vi "CCC Example - Client.vi"() -> ()   [LabVIEW 2010]
doc: "This VI shows an example of how to use the CVT Client Communication API. This VI is meant to be used in conjunction with \"CCC Server Example.vi\"."
uses:
  vi.lib/NI/CCC/Tag Configuration.ctl
  <vilib>/NI/Current Value Table/Type Defs/Data Types.ctl
  vi.lib/NI/CCC/Tag Direction.ctl
  <vilib>/NI/Current Value Table/Type Defs/Single Tag.ctl
  <vilib>/NI/Current Value Table/Type Defs/File Format.ctl
  <vilib>/NI/Current Value Table/Type Defs/Tag Grouping set.ctl
  <vilib>/NI/Current Value Table/DataTypes/Double_Write.vi
  <vilib>/NI/Current Value Table/DataTypes/String_Write.vi
  <vilib>/NI/Current Value Table/DataTypes/Double_Read.vi
  <vilib>/NI/Current Value Table/DataTypes/Boolean_Read.vi
  <vilib>/NI/Current Value Table/Type to Enum.vi
  <vilib>/NI/Current Value Table/DataTypes/Double_Type To Enum.vi
  <vilib>/NI/Current Value Table/DataTypes/String_Type To Enum.vi
  <vilib>/NI/Current Value Table/DataTypes/Boolean_Type To Enum.vi
  <vilib>/NI/Current Value Table/FGVs/CVT Globals.vi
  <vilib>/NI/Current Value Table/FGVs/Tag Memory.vi
  <vilib>/NI/Current Value Table/Memory Block.vi
  <vilib>/NI/Current Value Table/DataTypes/Double_Memory Block.vi
  <vilib>/NI/Current Value Table/DataTypes/String_Memory Block.vi
  <vilib>/NI/Current Value Table/DataTypes/Boolean_Memory Block.vi
  vi.lib/NI/CCC/NI_CCC.lvlib
  <vilib>/NI/Current Value Table/Current Value Table.lvlib
panel:
  in  "Tab Control":enum32{"Tag Configuration", "Program Operation"}(tab)=enum."Program Operation"
  in  "CVT Tags":T1[](array[typedef])=[{"Data Type"=enum."Double", "Name"="Input1", "Value"="", "Description"=""}, {"Data Type"=enum."Double", "Name"="Input2", "Value"="", "Description"=""}, {"Data Type"=enum."Double", "Name"="Output", "Value"="", "Description"=""}, {"Data Type"=enum."String", "Name"="Operation", "Value"="", "Description"=""}, {"Data Type"=enum."Boolean", "Name"="ClientError", "Value"="", "Description"=""}]
  in  "CCC Tags":T3[](array[typedef])=[{"name"="Input1", "data type"=enum."Double", "direction"=enum."Write", "bound address"="Float1"}, {"name"="Input2", "data type"=enum."Double", "direction"=enum."Write", "bound address"="Float2"}, {"name"="Output", "data type"=enum."Double", "direction"=enum."Read", "bound address"="Float3"}, {"name"="Operation", "data type"=enum."String", "direction"=enum."Write", "bound address"="Operand"}, {"name"="ClientError", "data type"=enum."Boolean", "direction"=enum."Read", "bound address"="Error"}]
  in  "Server IP Address":string="0.0.0.0"
  in  "Input1":dbl=4.0
  in  "Input2":dbl=2.0
  in  "Operation":string="Add" caption="Choose from:\nAdd, Subtract, Multiply, Divide"
  in  "stop":bool
  out "Output":dbl
  out "Error":bool
  # "Directions:\nRun \"CCC Example - Server.vi\" first, then run this VI."
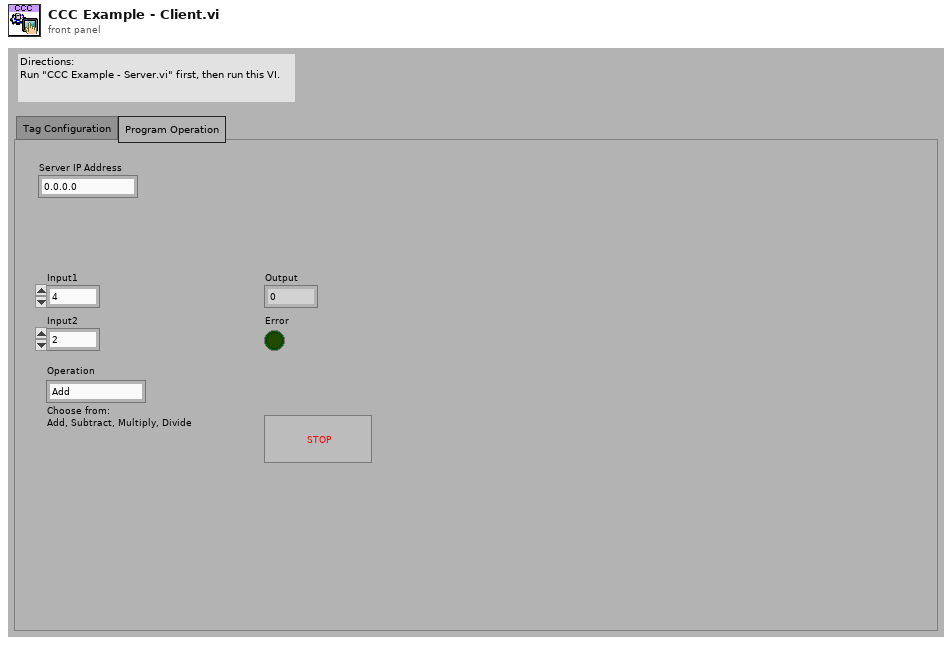
[diagram p1: front panel]
types:
  T1 = typedef "Current Value Table.lvlib/Single Tag.ctl" = cluster{"Data Type":T2, "Name":string, "Value":string, "Description":string}
  T2 = typedef "Current Value Table.lvlib/Data Types.ctl" = enum16{"Double", "Single", "I64", "I32", "I16", "I8", "U64", "U32", "U16", "U8", "String", "Boolean", "Array of U8", "Array of U16", "Array of U32", "Array of U64", "Array of I64", "Array of I32", "Array of I16", "Array of I8", "Array of Double", "Array of Single", "Array of Boolean", "Array of String"}
  T3 = typedef "NI_CCC.lvlib/Tag Configuration.ctl" = cluster{"name":string, "data type":T2, "direction":T4, "bound address":string}
  T4 = typedef "NI_CCC.lvlib/Tag Direction.ctl" = enum32{"<none>", "Read", "Write"}
  T5 = typedef "Current Value Table.lvlib/File Format.ctl" = cluster{"Tags":T1[], "Group Listings":T6[]}
  T6 = typedef "Current Value Table.lvlib/Tag Grouping set.ctl" = cluster{"Group":string, "Tag Names":string[]}
  T7 = typedef "NI_CCC.lvlib/Connection ID.ctl" = cluster{"server ID":string, "connection ID":T8, "meta data":T9[], "write tag list":T3[], "read tag list":T3[]}
  T8 = typedef "NI STM.lvlib/TCP Connection Info.ctl" = cluster{"connection ID":refnum<k5>, "Meta data":T9[]}
  T9 = typedef "NI STM.lvlib/MetaDataElement.ctl" = string
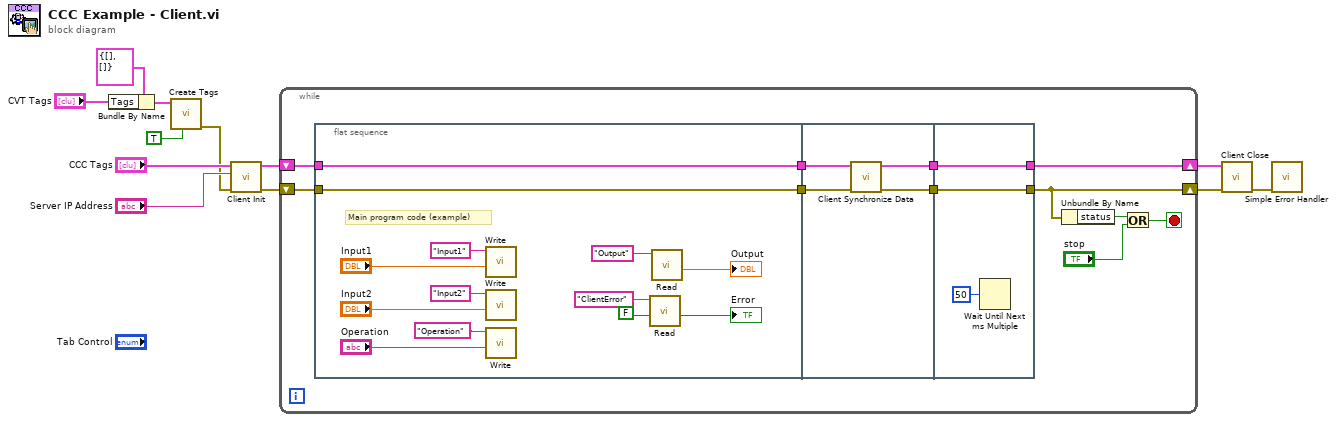
[diagram p0: block diagram]
diagram:
  n1 = Bundle By Name(cluster=T5 {"Tags"=[], "Group Listings"=[]} ("CVT Tags to Create"), "Tags"="CVT Tags") -> (w2:T5)
  n2 = call <vilib>:"Create Tags.vi"("Overwrite Duplicates? (F)"=TRUE, "CVT Tags to Create"=w2) -> ("error out"=w6:errorcluster)  [unwired: 9 in]
  n3 = call "Client Init.vi"("error in"=w6, "server IP address"="Server IP Address", "tag list"="CCC Tags") -> ("error out"=w7:errorcluster, "connection ID"=w12:T7)  [unwired: 7 in]
  n4 = while {
    shift-right: [w15] -> w9
    shift-left: w7 -> [w21]
    shift-right: [w19] -> w10
    shift-left: w12 -> [w23]
    stop <- w16 stop-if-true
    n5 = flat-sequence {
      tunnel: w23 -> [w36]
      tunnel: [w36] -> w22
      tunnel: w21 -> [w35]
      tunnel: [w35] -> w20
      tunnel: w22 -> [w40]
      tunnel: w20 -> [w39]
      tunnel: [w38] -> w18
      tunnel: [w37] -> w13
      tunnel: [w42] -> w19
      tunnel: [w41] -> w15
      tunnel: w18 -> [w41]
      tunnel: w13 -> [w42]
      frame #0 {
        # "Main program code (example)"
        n6 = call-poly <vilib>:"Write.vi"("Value"="Input1", "Tag Name"="Input1") -> ()  [unwired: 9 in, 1 out]
        n7 = call-poly <vilib>:"Write.vi"("Value"="Input2", "Tag Name"="Input2") -> ()  [unwired: 9 in, 1 out]
        n8 = call-poly <vilib>:"Write.vi"("Value"="Operation", "Tag Name"="Operation") -> ()  [unwired: 9 in, 1 out]
        n9 = call-poly <vilib>:"Read.vi"("Default"=FALSE, "Tag Name"="ClientError") -> ("Value"=→"Error":bool)  [unwired: 8 in, 1 out]
        n10 = call-poly <vilib>:"Read.vi"("Tag Name"="Output") -> ("Value"=→"Output":dbl)  [unwired: 9 in, 1 out]
      }
      frame #1 {
        n11 = call "Client Synchronize Data.vi"("error in"=w39, "connection ID in"=w40) -> ("error out"=w38:errorcluster, "connection ID out"=w37:T7)  [unwired: 8 in]
      }
      frame #2 {
        n12 = Wait Until Next ms Multiple(millisecond multiple=u32 50) -> ()  [unwired: 1 out]
      }
    }
    n13 = Unbundle By Name(w15) -> ("status"=w14:bool)
    n14 = Or(x=w14, y="stop") -> (x .or. y?=w16:bool)
  }
  n15 = call "Client Close.vi"("error in"=w9, "connection ID"=w10) -> ("error out"=w5:errorcluster)  [unwired: 9 in]
  n16 = call <vilib>:"Simple Error Handler.vi"("error in (no error)"=w5) -> ()  [unwired: 4 in, 5 out]
